vi "SwerveAccelerationSlewLimiting.vi"(9 "Joystick Y":dbl, 11 "Joystick X":dbl) -> ()   [LabVIEW 2020]
uses:
  GlobalDrivebase.vi
  GlobalPoseAndTargeting.vi
panel:
  in  "Deceleration Limt (ft/s^2)":dbl
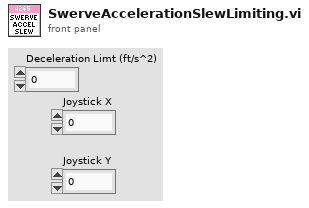
[diagram p1: front panel]
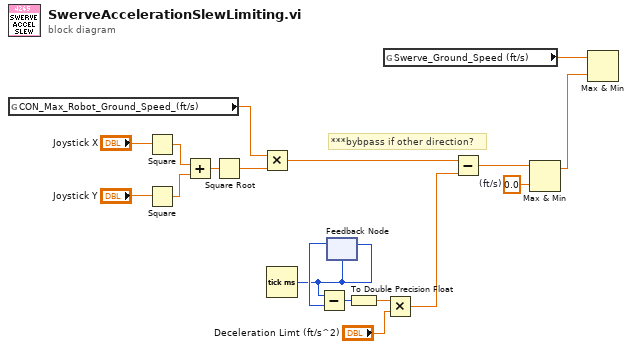
[diagram p0: block diagram]
diagram:
  w2 = 0.0  # (ft/s)
  # "***bybpass if other direction?"
  n1 = global read "GlobalDrivebase.vi" "CON_Max_Robot_Ground_Speed_(ft/s)"() -> (w12:dbl)
  n2 = Square(x="Joystick X") -> (x^2=w17:dbl)
  n3 = Square(x="Joystick Y") -> (x^2=w18:dbl)
  n4 = Add(x=w17, y=w18) -> (x+y=w16:dbl)
  n5 = Square Root(x=w16) -> (sqrt(x)=w13:dbl)
  n6 = Multiply(x=w12, y=w13) -> (x*y=w6:dbl)
  n7 = Tick Count (ms)() -> (millisecond timer value=w10:u32)
  n8 = feedback-in #1(w10) -> ()
  n9 = feedback #1(w10) -> (w11:u32)
  n10 = Subtract(x=w10, y=w11) -> (x-y=w9:u32)
  n11 = To Double Precision Float(number=w9) -> (double precision float=w8:dbl)
  n12 = global read "GlobalPoseAndTargeting.vi" "Swerve_Ground_Speed (ft/s)"() -> (w4:dbl)
  n13 = Multiply(x=w8, y="Deceleration Limt (ft/s^2)") -> (x*y=w5:dbl)
  n14 = Subtract(x=w6, y=w5) -> (x-y=w3:dbl)
  n15 = Max & Min(x=w3, y=w2) -> (max(x,y)=w1:dbl)  [unwired: 1 out]
  n16 = Max & Min(x=w4, y=w1) -> ()  [unwired: 2 out]
